vi "Lezeti_Power_Monitor_33_g.vi"() -> ()   [LabVIEW 2014]
uses:
  <vilib>/measure/madcrms.llb/Basic Averaged DC-RMS for N Chan.vi
  <vilib>/measure/madcrms.llb/Basic Averaged DC-RMS for 1 Chan.vi
  <vilib>/Utility/file.llb/Write To Spreadsheet File (DBL).vi
  <vilib>/measure/NI_MAPro.lvlib
panel:
  out "DC Current (Amps)":dbl
  out "DC Voltage":dbl
  out "DC Power (Watts)":dbl
  out "Power Factor":dbl
  in  "Average Power Output File":path
  out "Run Date":string
  out "Run Time":string
  out "Elapsed Time (s)":dbl
  out "Apparent Power (VA)":dbl
  out "Average Power (Watts)":dbl
  out "Instantaneous Power Waveform":waveform(dbl)[](graph)
  out "RMS Voltage L1-L2":dbl
  out "L1 RMS Current":dbl
  in  "Burden Resistor (ohms) (1000)":dbl
  in  "CT Ratio (Iout/Iin) (.0003332)":dbl
  in  "Acquire Sample Size (1000)":dbl
  in  "Acquire Rate (Hz) (1000)":dbl
  in  "Acquire Timeout (1000)":dbl
  out "Line 1 Current Waveform":waveform(dbl)[](graph)
  out "Voltage L1-L2":waveform(dbl)[](graph)
  in  "stop":bool
  # "For Lezeti Air Conditioning System (Greenpath Tech)\nBy Matsu Thornton\nJuly 2016"
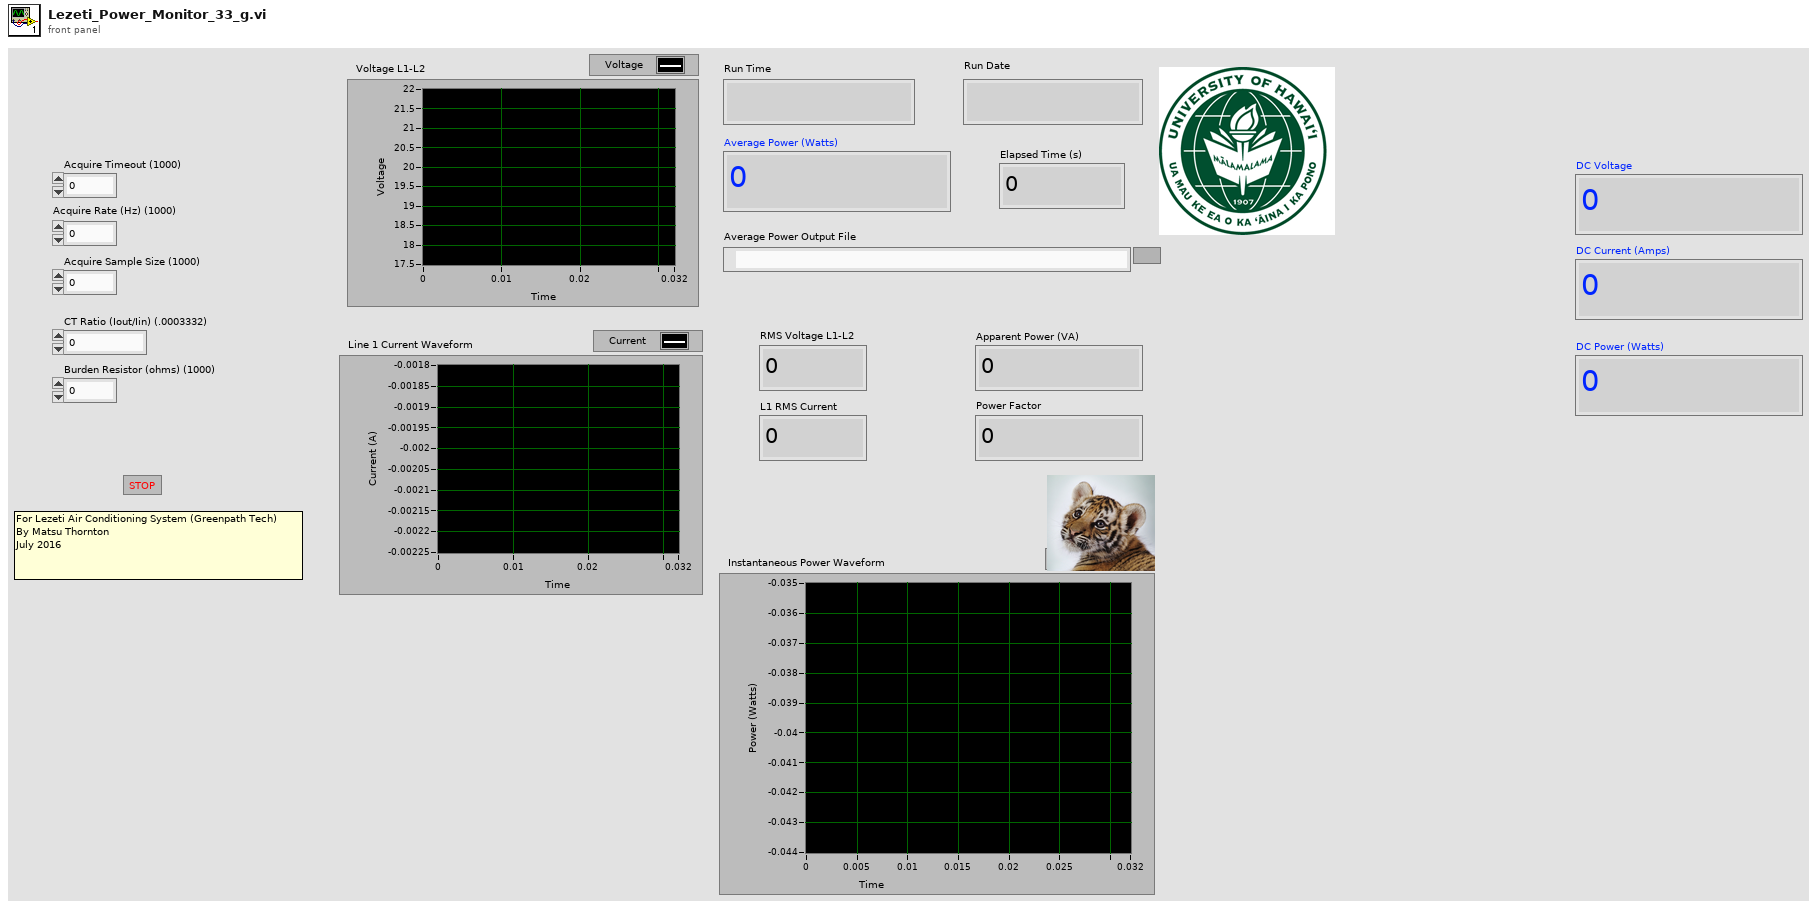
[diagram p1: front panel]
types:
  T1 = typedef "NI_Matrix.lvlib/RealMatrix.ctl" = dbl[][]
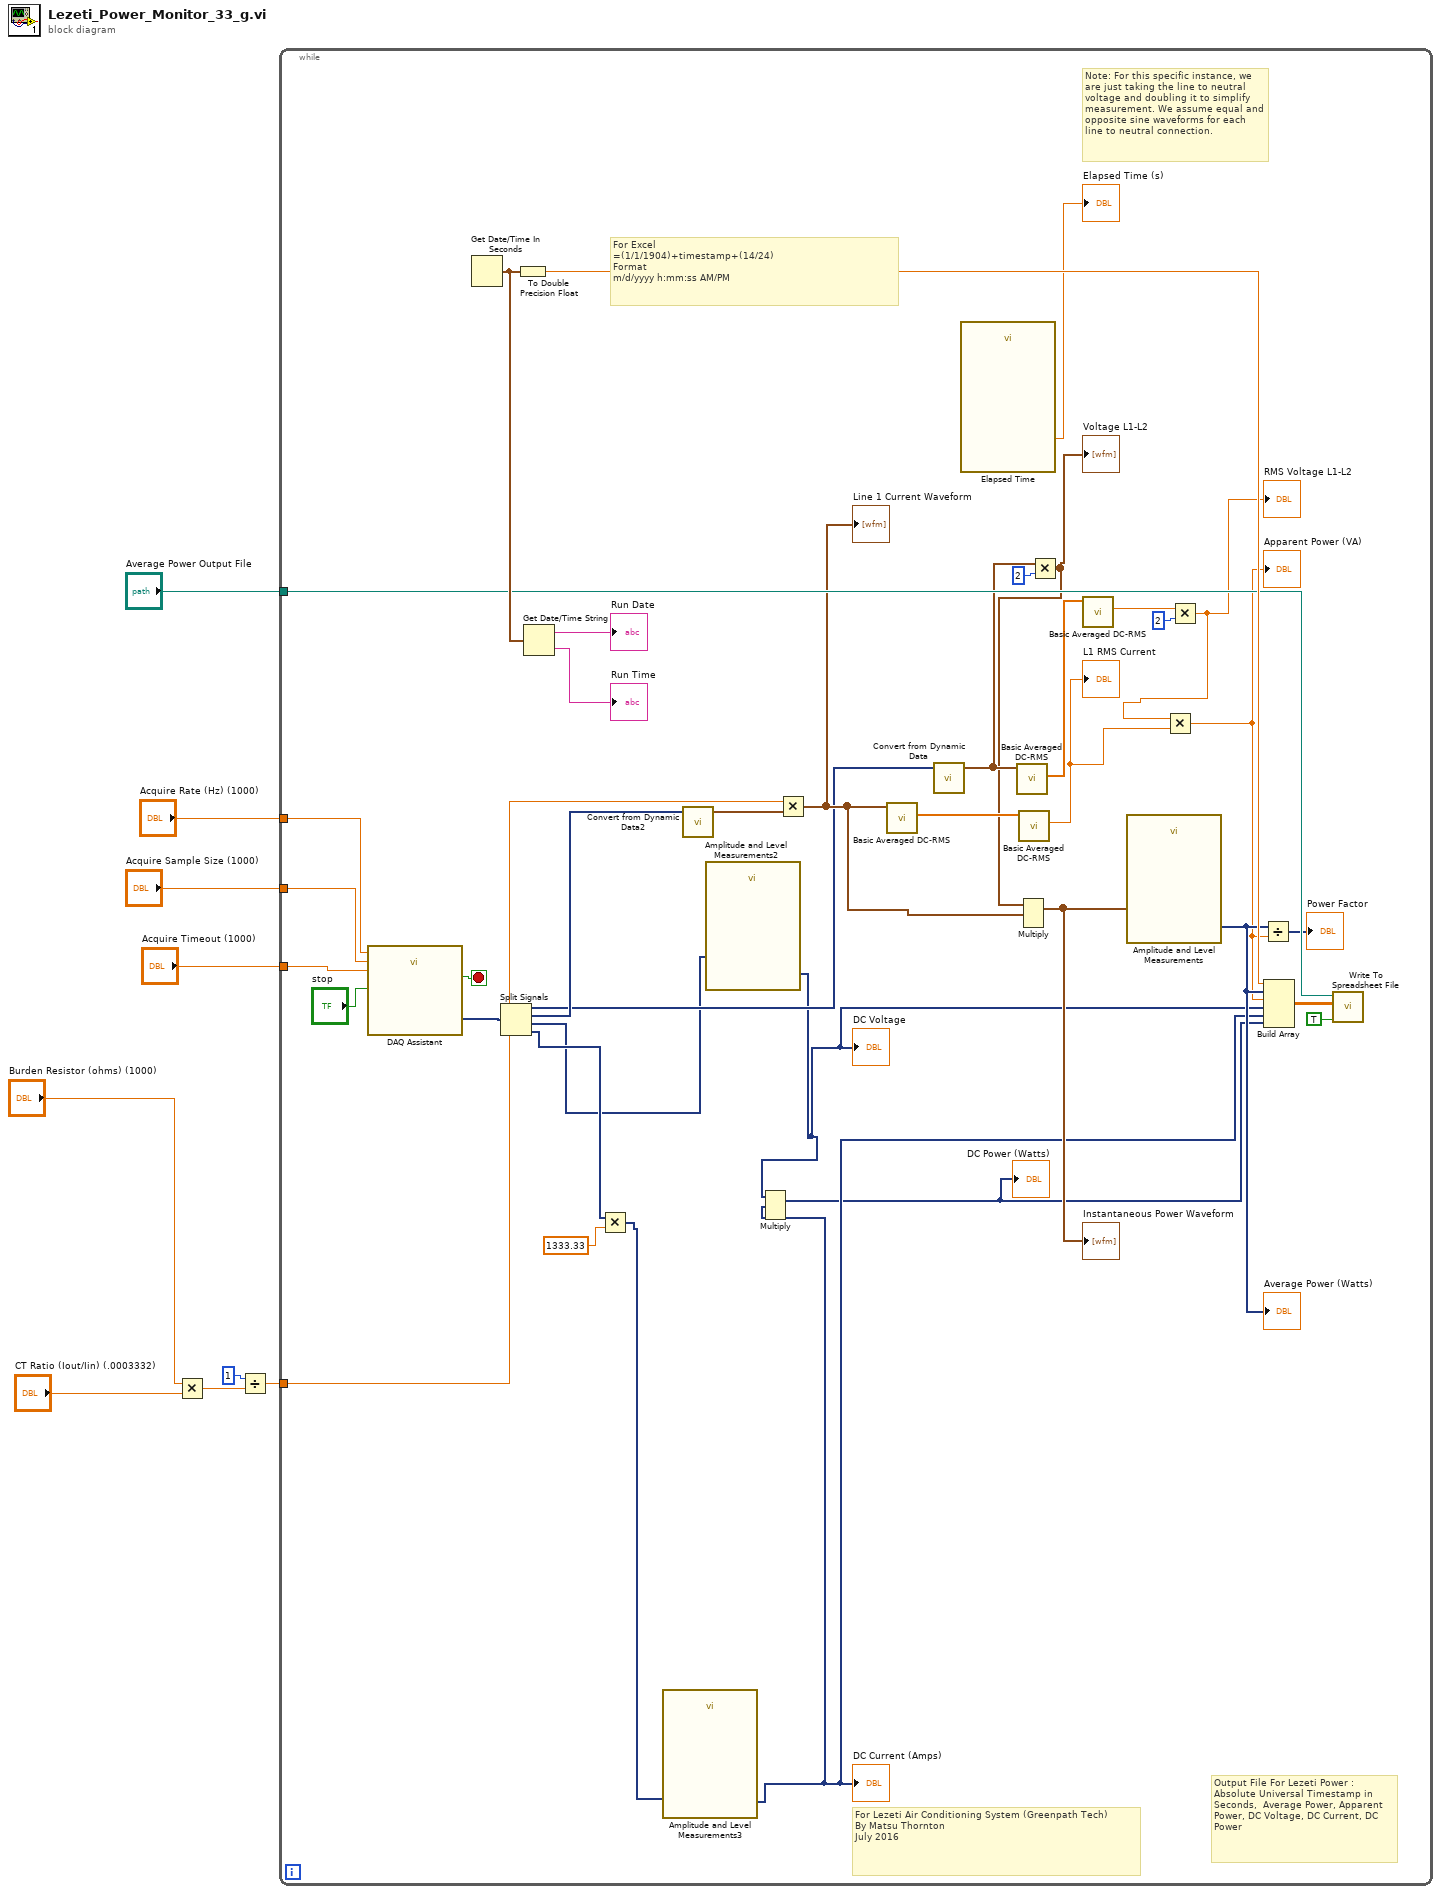
[diagram p0: block diagram]
diagram:
  n1 = Multiply(x="Burden Resistor (ohms) (1000)", y="CT Ratio (Iout/Iin) (.0003332)") -> (x*y=w3:dbl)
  n2 = Divide(x=1, y=w3) -> (x/y=w2:dbl)
  n3 = while {
    tunnel: "Acquire Timeout (1000)" -> [w15]
    tunnel: "Acquire Rate (Hz) (1000)" -> [w17]
    tunnel: "Acquire Sample Size (1000)" -> [w16]
    tunnel: w2 -> [w26]
    tunnel: "Average Power Output File" -> [w37]
    stop <- w34 stop-if-true
    # "Output File For Lezeti Power :\nAbsolute Universal Timestamp in Seconds,  Average Power, Apparent Power, DC Voltage, DC Current, DC Power"
    # "Note: For this specific instance, we are just taking the line to neutral voltage and doubling it to simplify measurement. We assume equal and opposite sine waveforms for each line to neutral connection."
    # "For Excel\n=(1/1/1904)+timestamp+(14/24)\nFormat\nm/d/yyyy h:mm:ss AM/PM"
    # "For Lezeti Air Conditioning System (Greenpath Tech)\nBy Matsu Thornton\nJuly 2016"
    n4 = call "DAQ Assistant"("rate"=w17, "number of samples"=w16, "timeout (s)"=w15, "stop (F)"="stop") -> ("data"=w28:dynamicdata, "stopped"=w34:bool)  [unwired: 12 in, 2 out]
    n5 = Get Date/Time In Seconds() -> (seconds since 1Jan1904=w41:timestamp)
    n6 = Split Signals(w28) -> (w19:dynamicdata, w27:dynamicdata, w10:dynamicdata, w11:dynamicdata)  [unwired: 4 in]
    n7 = To Double Precision Float(number=w41) -> (double precision float=w42:dbl)
    n8 = Get Date/Time String(seconds (now)=w41) -> (date string=→"Run Date":string, time string=→"Run Time":string)  [unwired: 2 in]
    n9 = Multiply(x=w11, y=1333.33) -> (x*y=w13:dynamicdata)
    n10 = call "Amplitude and Level Measurements3"("Signals"=w13) -> ("Mean (DC)"=w25:dynamicdata)  [unwired: 13 in, 1 out]
    "DC Current (Amps)" <- w25
    n11 = call "Convert from Dynamic Data2"("Dynamic Data Type"=w27) -> ("Array of Waveform"=w46:waveform(dbl)[])  [unwired: 3 in]
    n12 = call "Amplitude and Level Measurements2"("Signals"=w10) -> ("Mean (DC)"=w12:dynamicdata)  [unwired: 13 in, 1 out]
    "DC Voltage" <- w12
    n13 = Multiply(1:w25, 2:w12) -> (0:w24:dynamicdata)  [unwired: 1 in, 1 out]
    "DC Power (Watts)" <- w24
    n14 = Multiply(x=w26, y=w46) -> (x*y=w22:waveform(dbl)[])
    "Line 1 Current Waveform" <- w22
    n15 = call-poly <vilib>:"Basic Averaged DC-RMS.vi"("signals in"=w22) -> ("RMS values"=w47:dbl[])  [unwired: 7 in, 3 out]
    n16 = call "Convert from Dynamic Data"("Dynamic Data Type"=w19) -> ("Array of Waveform"=w29:waveform(dbl)[])  [unwired: 3 in]
    n17 = call "Elapsed Time"() -> ("Elapsed Time (s)"=→"Elapsed Time (s)":dbl)  [unwired: 12 in, 7 out]
    n18 = call-poly <vilib>:"Basic Averaged DC-RMS.vi"("signals in"=w29) -> ("RMS values"=w48:dbl[])  [unwired: 7 in, 3 out]
    n19 = call-poly <vilib>:"Basic Averaged DC-RMS.vi"("signal in"=w47) -> ("RMS value"=w21:dbl)  [unwired: 7 in, 3 out]
    "L1 RMS Current" <- w21
    n20 = Multiply(x=w29, y=2) -> (x*y=w18:waveform(dbl)[])
    "Voltage L1-L2" <- w18
    n21 = Multiply(1:w22, 2:w18) -> (0:w45:waveform(dbl)[])  [unwired: 1 in, 1 out]
    "Instantaneous Power Waveform" <- w45
    n22 = call-poly <vilib>:"Basic Averaged DC-RMS.vi"("signal in"=w48) -> ("RMS value"=w31:dbl)  [unwired: 7 in, 3 out]
    n23 = call "Amplitude and Level Measurements"("Signals"=w45) -> ("Mean (DC)"=w36:dynamicdata)  [unwired: 13 in, 1 out]
    "Average Power (Watts)" <- w36
    n24 = Multiply(x=w31, y=2) -> (x*y=w20:dbl)
    "RMS Voltage L1-L2" <- w20
    n25 = Multiply(x=w20, y=w21) -> (x*y=w33:dbl)
    "Apparent Power (VA)" <- w33
    n26 = Divide(x=w36, y=w33) -> (x/y=→"Power Factor":dynamicdata)
    n27 = Build Array(w42, w36, w33, w12, w25, w24) -> (w43:T1)
    n28 = call-poly <vilib>:"Write To Spreadsheet File.vi"("append to file? (new file:F)"=TRUE, "2D data"=w43, "file path (dialog if empty)"=w37) -> ()  [unwired: 5 in, 1 out]
  }
